vi "create_report.vi"(8 "error in (no error)":errorcluster, 11 "ReportService in":refnum<class "ReportService.lvclass">) -> (0 "error out":errorcluster, 3 "ReportService out":refnum<class "ReportService.lvclass">)   [LabVIEW 2024, in "ReportService.lvclass"]
uses:
  ReportService.lvclass
  ReportService.lvclass/ReportService.ctl
  PDFStudentReport/PDFStudentReport.lvclass
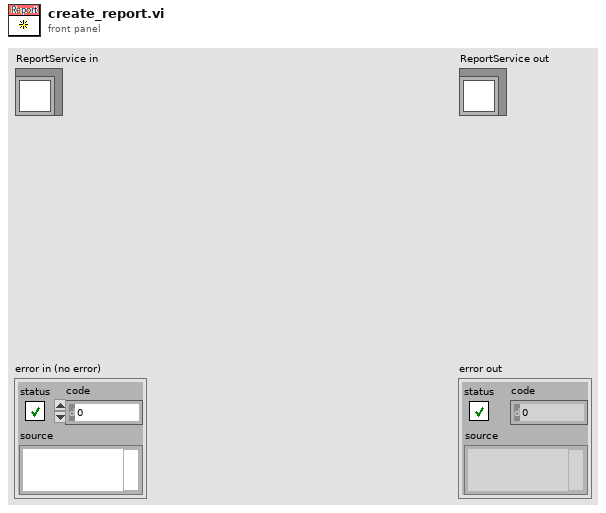
[diagram p1: front panel]
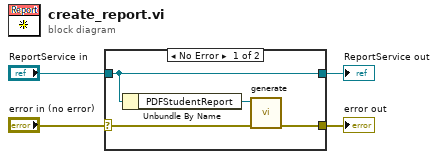
[diagram p0: block diagram]
diagram:
  n1 = case shown="No Error" "error in (no error)" {
    selector: "error in (no error)" -> [w6 w10]
    tunnel: [w5 w10] -> w3
    tunnel: [w8 w9] -> w1
    tunnel: "ReportService in" -> [w8 w9]
    frame No Error {
      n2 = Unbundle By Name(w8) -> ("PDFStudentReport"=w7:refnum<class "PDFStudentReport.lvclass">)
      n3 = call-dynamic "generate.vi"("error in (no error)"=w6, "PDFStudentReport in"=w7) -> ("error out"=w5:errorcluster)  [unwired: 8 in, 1 out]
    }
    frame Error {
    }
  }
  "error out" <- w3
  "ReportService out" <- w1
